vi "PCert-ConfigPageNF-InitializeDBActor.vi"(9 "FTW Actor Instance Configuration":string="{\n  \"Identity\": \"ActorName\",\n  \"InboxAddress\": \"tcp://127.0.0.1:*\",\n  \"PublisherAddress\": \"tcp://127.0.0.1:*\",\n  \"DebugEnableInboxLogging\": false,\n  \"DebugEnableJobLogging\": false,\n  \"DebugShowPanel\": false\n}", 10 "Initialization Job Sequence":string, 11 "ERP-ConfigPageNF.lvclass":refnum<class "PCert-ConfigPageNF.lvclass">) -> (0 "error out":errorcluster, 3 "ERP-ConfigPageNF out":refnum<class "PCert-ConfigPageNF.lvclass">)   [LabVIEW 2013, in "PCert-ConfigPageNF.lvclass"]
uses:
  PCert-ConfigPageNF.lvclass
  PCert-ConfigPageNF.lvclass/PCert-ConfigPageNF.ctl
  ftw-dataflow/Actor/src/Connector/FTW-ActorConnector.lvclass
  ftw-dataflow/Core/src/Reflection/FTW-Reflection-Type.vi
  ftw-dataflow/Core/src/JSON/FTW-JSON-Core-LibraryFilepath.vi
  ftw-dataflow/Core/src/JSON/FTW-JSON-Core-GetFlattenedValue.vi
  ftw-dataflow/Core/src/JSON/FTW-JSON-Core-LibraryError.vi
  ftw-dataflow/Core/utils/CodeGen/JSON Deserialize/FTW-JSON-Deserialize.xnode
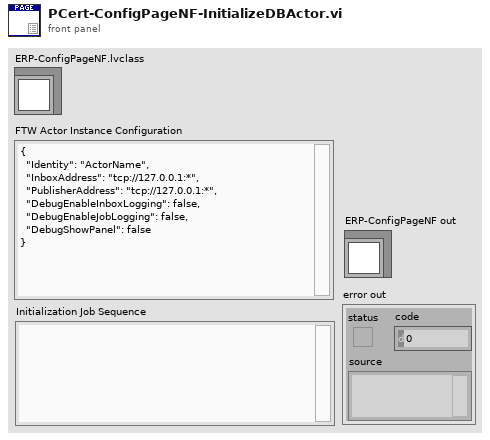
[diagram p1: front panel]
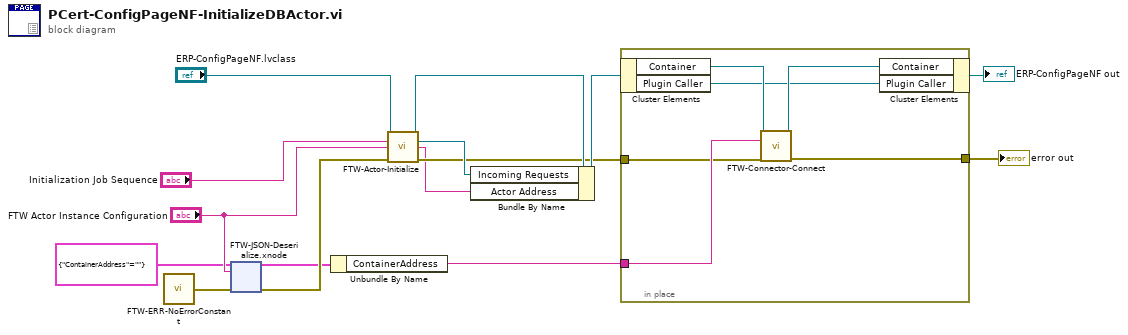
[diagram p0: block diagram]
diagram:
  n1 = call "FTW-ERR-NoErrorConstant.vi"() -> ("no error"=w13:errorcluster)
  n2 = xnode "FTW-JSON-Deserialize.xnode"("Type and Defaults"=cluster{"ContainerAddress":string} {"ContainerAddress"=""}, "JSON String"="FTW Actor Instance Configuration", "error in"=w13) -> ("Values"=w1:cluster{"ContainerAddress":string}, "error out"=w12:errorcluster)
  n3 = Unbundle By Name(w1) -> ("ContainerAddress"=w8:string)
  n4 = call-dynamic "FTW-Actor-Initialize.vi"("FTW Actor Instance Type"="ERP-ConfigPageNF.lvclass", "Initialization Job Sequence"="Initialization Job Sequence", "Actor Instance Configuration"="FTW Actor Instance Configuration", "error in"=w12) -> ("FTW Actor Instance"=w10:refnum<class "PCert-ConfigPageNF.lvclass">, "Incoming Requests"=w11:refnum<event-registration>, "Actual Server Address"=w4:string, "error out"=w7:errorcluster)  [unwired: 8 in]
  n5 = Bundle By Name(cluster=w10, "Incoming Requests"=w11, "Actor Address"=w4) -> (w9:refnum<class "PCert-ConfigPageNF.lvclass">)
  n6 = in-place {
    in-place-border: w8 -> [w20]
    in-place-border: w7 -> [w19]
    in-place-border: [w17] -> w3
    n7 = in-place-cluster #1(w9) -> ("Container"=w21:refnum<class "FTW-ActorConnector.lvclass">, "Plugin Caller"=w16:refnum<class "FTW-ActorConnector.lvclass">)
    n8 = call-dynamic "FTW-Connector-Connect.vi"("FTW Actor Connector Type"=w21, "Instance Inbox Address"=w20, "error in"=w19) -> ("FTW Actor Connector"=w18:refnum<class "FTW-ActorConnector.lvclass">, "error out"=w17:errorcluster)  [unwired: 11 in]
    n9 = in-place-cluster #1("Container"=w18, "Plugin Caller"=w16) -> (→"ERP-ConfigPageNF out":refnum<class "PCert-ConfigPageNF.lvclass">)
  }
  "error out" <- w3
